vi "svfa_Check Waveform Parameter Continuity (1xM) [Dual FFT].vi"(0 "stimulus signals X [EUx]":waveform(dbl)[](array[waveform]), 1 "restart averaging (F)":bool, 5 "response signal Y [EUy]":waveform(dbl), 7 "checks for channel parameter change":T1, 9 "checks for multichannel parameters":T2, 11 "error in":errorcluster) -> (4 "dup stimulus signals X [EUx]":waveform(dbl)[](array[waveform]), 6 "dup response signal Y [EUy]":waveform(dbl), 8 "waveform parameter changed":bool, 10 "multichannel parameter changed":bool, 15 "error out":errorcluster)   [LabVIEW 2017]
uses:
  <vilib>/addons/_NISVFA/_Shared subVIs/Common/svc_Check for Waveform Parameter Continuity (no state).vi
  <vilib>/addons/_NISVFA/_Shared subVIs/Common/svc_Get SV Channel Info.vi
  <vilib>/addons/_NISVFA/_Shared subVIs/Common/svc_Engineering Units to Unit Label.vi
  <vilib>/addons/_NISVFA/_Shared subVIs/Common/svc_Unit Label to Engineering Units.vi
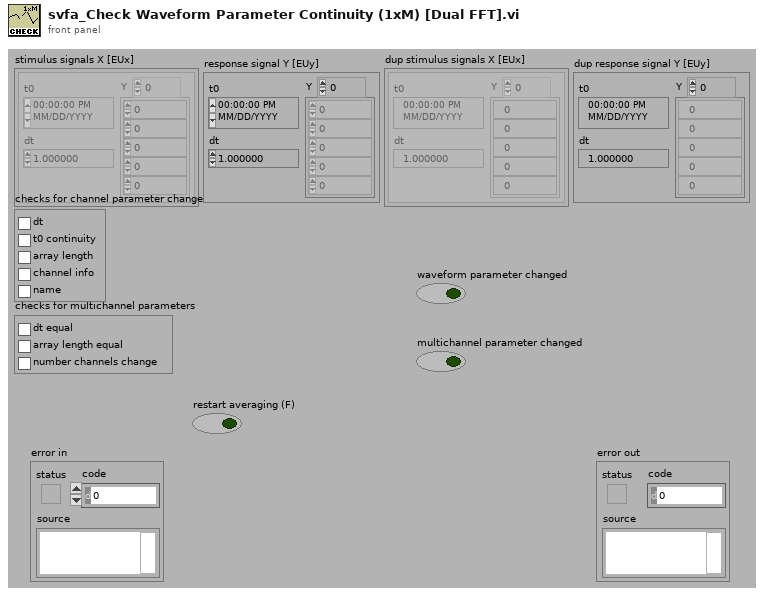
[diagram p1: front panel]
types:
  T1 = cluster{"dt":bool, "t0 continuity":bool, "array length":bool, "channel info":bool, "name":bool}
  T2 = cluster{"dt equal":bool, "array length equal":bool, "number channels change":bool}
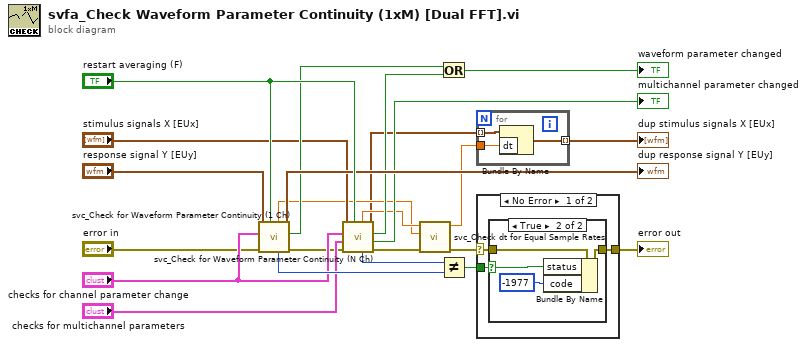
[diagram p0: block diagram]
diagram:
  n1 = call <vilib>:"svc_Check for Waveform Parameter Continuity (1 Ch).vi"("restart averaging (F)"="restart averaging (F)", "error in (no error)"="error in", "checks for channel parameter change"="checks for channel parameter change", "scaled signal [EU]"="response signal Y [EUy]") -> ("error out"=w19:errorcluster, "waveform parameter changed"=w14:bool, "dup scaled signal [EU]"=→"dup response signal Y [EUy]":waveform(dbl), "array length"=w23:i32, "dt"=w8:dbl)  [unwired: 2 in, 1 out]
  n2 = call <vilib>:"svc_Check for Waveform Parameter Continuity (N Ch).vi"("restart averaging (F)"="restart averaging (F)", "error in (no error)"=w19, "checks for multichannel parameters"="checks for multichannel parameters", "checks for channel parameter change"="checks for channel parameter change", "scaled signal(s)"="stimulus signals X [EUx]") -> ("error out"=w7:errorcluster, "multichannel parameter changed"=→"multichannel parameter changed":bool, "waveform parameter changed"=w15:bool, "dup scaled signal(s)"=w3:waveform(dbl)[], "array length"=w22:i32, "dt"=w9:dbl)  [unwired: 1 out]
  n3 = call <vilib>:"svc_Check dt for Equal Sample Rates.vi"("error in (no error)"=w7, "dt Y"=w8, "dt X"=w9) -> ("error out"=w6:errorcluster, "dt Y"=w1:dbl)  [unwired: 7 in]
  n4 = Or(x=w14, y=w15) -> (x .or. y?=→"waveform parameter changed":bool)
  n5 = Not Equal?(x=w22, y=w23) -> (x != y?=w5:bool)
  n6 = for {
    tunnel: w3 -> [w26] mode=indexing
    tunnel: [w25] -> w2 mode=indexing
    tunnel: w1 -> [w24]
    n7 = Bundle By Name ("Build Waveform")(cluster=w26, "dt"=w24) -> (w25:waveform(dbl))
  }
  "dup stimulus signals X [EUx]" <- w2
  n8 = case shown="No Error" w6 {
    selector: w6 -> [w28 w35]
    tunnel: w5 -> [w29 _]
    tunnel: [w27 w35] -> w4
    frame No Error {
      n9 = case shown="True" w29 {
        selector: w29 -> [_ w32]
        tunnel: [w30 w34] -> w27
        tunnel: w28 -> [w30 w31]
        frame False {
        }
        frame True {
          n10 = Bundle By Name(cluster=w31, "status"=w32, "code"=-1977) -> (w34:errorcluster)
        }
      }
    }
    frame Error {
    }
  }
  "error out" <- w4
